vi "fit function selector.vi"(6 "fit using":T1=enum."varshni", 10 "temperature":dbl[](array[numeric]), 11 "best fit parameters":dbl[](array[numeric])) -> (0 "fit function name":string="varshni fit function.vi", 1 "vi reference":T2, 2 "freq out":dbl[](array[numeric]))   [LabVIEW 2018]
uses:
  <vilib>/gmath/NumericalOptimization/LM model function reference.ctl
  fit function selector control.ctl
  <vilib>/gmath/NI_Gmath.lvlib
panel:
  in  "mode":enum16{"empty", "write", "read"}(ring)=enum."write"
  out "best fit params out":dbl[](array[numeric])
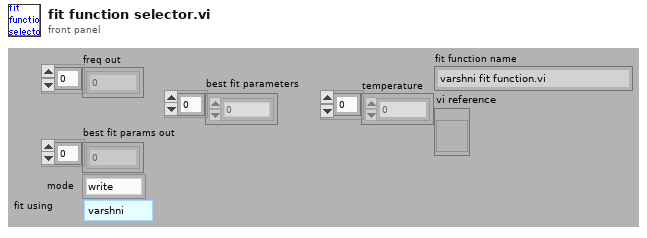
[diagram p1: front panel]
types:
  T1 = typedef "fit function selector control.ctl" = enum16{"linear", "varshni", "varshni5", "LogMinusT", "hyperbola", "einstein", "sine", "sine2theta", "cos2theta"}
  T2 = typedef "NI_Gmath.lvlib/LM model function reference.ctl" = refnum<vi>
  T3 = cluster{"file name":string, "a":dbl, "b":dbl, "c":dbl, "comment":string}
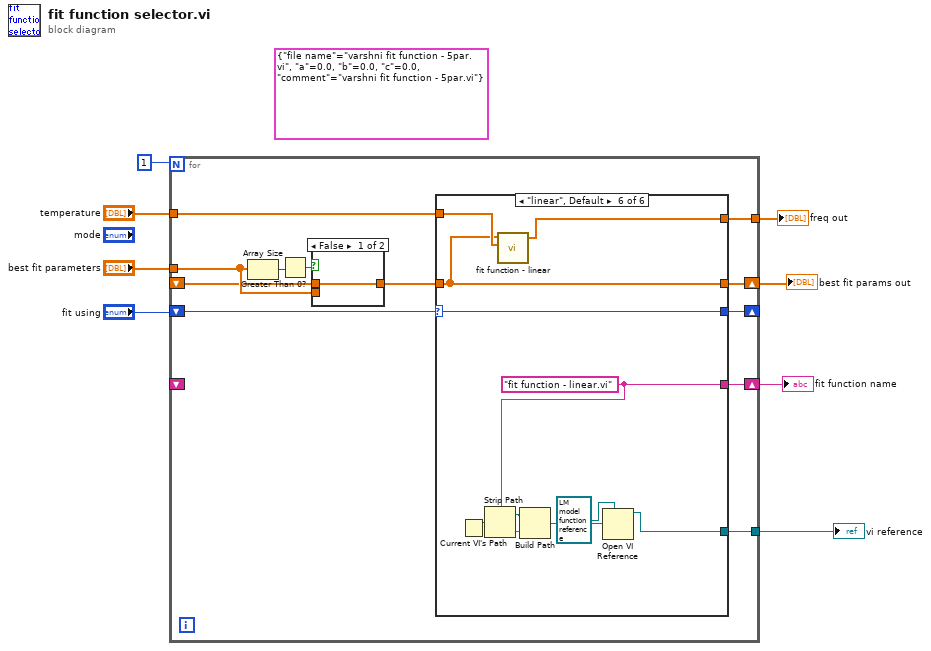
[diagram p0: block diagram]
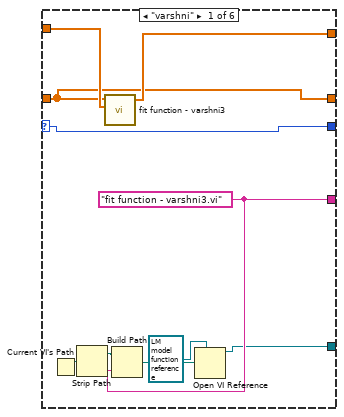
[diagram p3: hidden frame]
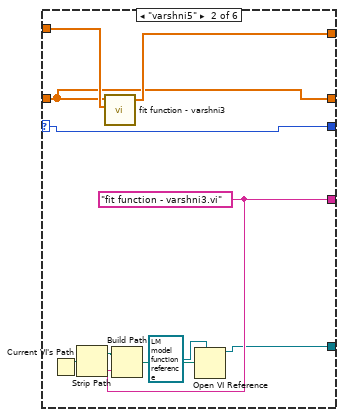
[diagram p4: hidden frame]
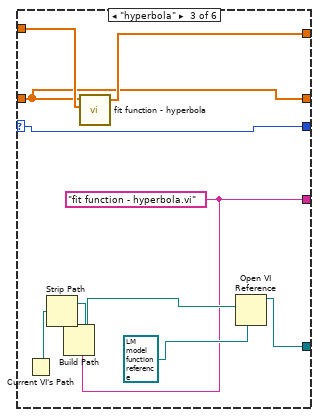
[diagram p5: hidden frame]
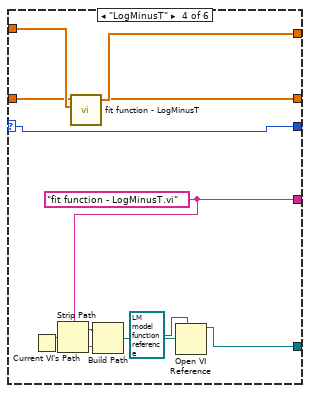
[diagram p6: hidden frame]
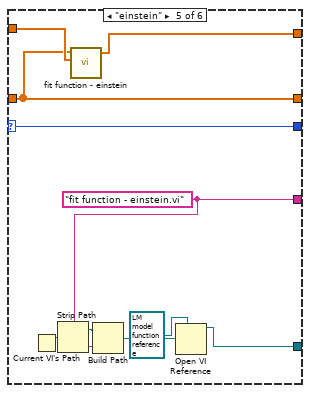
[diagram p7: hidden frame]
diagram:
  (unwired) T3 {"file name"="varshni fit function - 5par.vi", "a"=0.0, "b"=0.0, "c"=0.0, "comment"="varshni fit function - 5par.vi"}
  n1 = for {
    N: 1 -> [_]
    tunnel: "temperature" -> [w20]
    tunnel: [w19] -> w7
    shift-right: [w16] -> w5
    shift-left: _ -> [w12]
    shift-right: [w10] -> _
    shift-left: "fit using" -> [w17]
    shift-right: [w18] -> w6
    shift-left: _ -> [_]
    tunnel: "best fit parameters" -> [w13]
    tunnel: [w9] -> w2
    n2 = Array Size(array=w13) -> (size(s)=w15:i32)
    n3 = Greater Than 0?(x=w15) -> (x > 0?=w14:bool)
    n4 = case shown="False" w14 {
      tunnel: [w21 w22] -> w11
      tunnel: w13 -> [_ w22]
      tunnel: w12 -> [w21 _]
      frame False {
      }
      frame True {
      }
    }
    n5 = case shown="\"linear\", Default" w17 {
      selector: w17 -> [w29 w39 w49 w59 w69 w79]
      tunnel: w11 -> [w30 w40 w50 w60 w70 w80]
      tunnel: w20 -> [w32 w42 w52 w62 w72 w82]
      tunnel: [w31 w41 w51 w61 w71 w81] -> w19
      tunnel: [w24 w34 w44 w54 w64 w74] -> w18
      tunnel: [w30 w40 w50 w60 w70 w80] -> w16
      tunnel: [w29 w39 w49 w59 w69 w79] -> w10
      tunnel: [w23 w33 w43 w53 w63 w73] -> w9
      frame "varshni" {
        w24 = "fit function - varshni3.vi" ("f(x,a) VI name Complex")
        n6 = Current VI's Path() -> (path=w27:path)
        n7 = Strip Path(path=w27) -> (stripped path=w28:path)  [unwired: 1 out]
        n8 = call "fit function - varshni3.vi"("X"=w32, "a"=w30) -> ("f(X,a)"=w31:dbl[])  [unwired: 2 in, 2 out]
        n9 = Build Path(base path=w28, name or relative path=w24) -> (appended path=w25:path)
        n10 = Open VI Reference(type specifier VI Refnum (for type only)=T2 refnum ("f(x,a)"), vi path=w25) -> (vi reference=w23:T2)  [unwired: 1 in, 4 out]
      }
      frame "varshni5" {
        w34 = "fit function - varshni3.vi" ("f(x,a) VI name Complex")
        n11 = Current VI's Path() -> (path=w37:path)
        n12 = Strip Path(path=w37) -> (stripped path=w38:path)  [unwired: 1 out]
        n13 = call "fit function - varshni3.vi"("X"=w42, "a"=w40) -> ("f(X,a)"=w41:dbl[])  [unwired: 2 in, 2 out]
        n14 = Build Path(base path=w38, name or relative path=w34) -> (appended path=w35:path)
        n15 = Open VI Reference(type specifier VI Refnum (for type only)=T2 refnum ("f(x,a)"), vi path=w35) -> (vi reference=w33:T2)  [unwired: 1 in, 4 out]
      }
      frame "hyperbola" {
        w44 = "fit function - hyperbola.vi" ("f(x,a) VI name Complex")
        n16 = Current VI's Path() -> (path=w47:path)
        n17 = Strip Path(path=w47) -> (stripped path=w48:path)  [unwired: 1 out]
        n18 = Build Path(base path=w48, name or relative path=w44) -> (appended path=w45:path)
        n19 = call "fit function - hyperbola.vi"("X"=w52, "a"=w50) -> ("f(X,a)"=w51:dbl[])  [unwired: 2 in, 2 out]
        n20 = Open VI Reference(type specifier VI Refnum (for type only)=T2 refnum ("f(x,a)"), vi path=w45) -> (vi reference=w43:T2)  [unwired: 1 in, 4 out]
      }
      frame "LogMinusT" {
        w54 = "fit function - LogMinusT.vi" ("f(x,a) VI name Complex")
        n21 = Current VI's Path() -> (path=w57:path)
        n22 = Strip Path(path=w57) -> (stripped path=w58:path)  [unwired: 1 out]
        n23 = call "fit function - LogMinusT.vi"("X"=w62, "a"=w60) -> ("f(X,a)"=w61:dbl[])  [unwired: 2 in, 2 out]
        n24 = Build Path(base path=w58, name or relative path=w54) -> (appended path=w55:path)
        n25 = Open VI Reference(type specifier VI Refnum (for type only)=T2 refnum ("f(x,a)"), vi path=w55) -> (vi reference=w53:T2)  [unwired: 1 in, 4 out]
      }
      frame "einstein" {
        w64 = "fit function - einstein.vi" ("f(x,a) VI name Complex")
        n26 = Current VI's Path() -> (path=w67:path)
        n27 = Strip Path(path=w67) -> (stripped path=w68:path)  [unwired: 1 out]
        n28 = call "fit function - einstein.vi"("X"=w72, "a"=w70) -> ("f(X,a)"=w71:dbl[])  [unwired: 2 in, 2 out]
        n29 = Build Path(base path=w68, name or relative path=w64) -> (appended path=w65:path)
        n30 = Open VI Reference(type specifier VI Refnum (for type only)=T2 refnum ("f(x,a)"), vi path=w65) -> (vi reference=w63:T2)  [unwired: 1 in, 4 out]
      }
      frame "linear", Default {
        w74 = "fit function - linear.vi" ("f(x,a) VI name Complex")
        n31 = Current VI's Path() -> (path=w77:path)
        n32 = Strip Path(path=w77) -> (stripped path=w78:path)  [unwired: 1 out]
        n33 = call "fit function - linear.vi"("X"=w82, "a"=w80) -> ("f(X,a)"=w81:dbl[])  [unwired: 2 in, 2 out]
        n34 = Build Path(base path=w78, name or relative path=w74) -> (appended path=w75:path)
        n35 = Open VI Reference(type specifier VI Refnum (for type only)=T2 refnum ("f(x,a)"), vi path=w75) -> (vi reference=w73:T2)  [unwired: 1 in, 4 out]
      }
    }
  }
  "freq out" <- w7
  "fit function name" <- w6
  "best fit params out" <- w5
  "vi reference" <- w2
